vi "Operation DVR.vi"(8 "Error In":errorcluster, 11 "DVR In":refnum<data-value>) -> (0 "Error Out":errorcluster, 2 "C":dbl, 3 "DVR Out":refnum<data-value>)   [LabVIEW 2023, in "Arithemetic Operation.lvclass"]
uses:
  Arithemetic Operation.lvclass
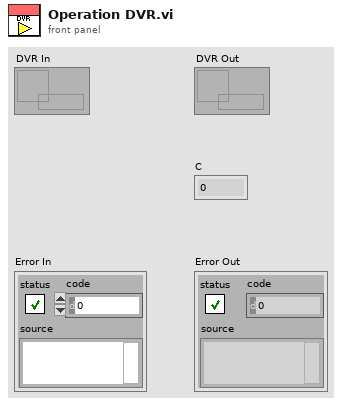
[diagram p1: front panel]
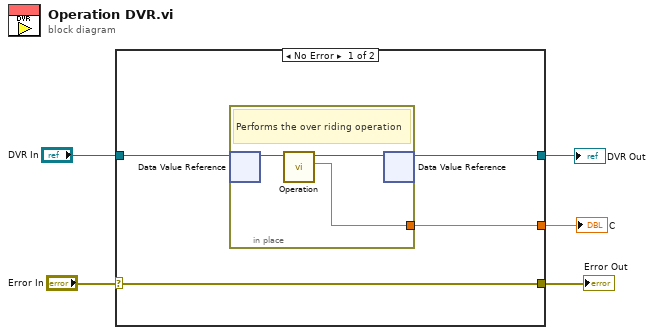
[diagram p0: block diagram]
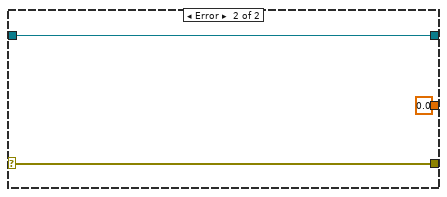
[diagram p2: hidden frame]
diagram:
  n1 = case shown="No Error" "Error In" {
    selector: "Error In" -> [w9 w15]
    tunnel: [w9 w15] -> w4
    tunnel: [w7 w14] -> w3
    tunnel: "DVR In" -> [w8 w14]
    tunnel: [w6 0.0 ("C")] -> w1
    frame No Error {
      n2 = in-place {
        in-place-border: [w10] -> w6
        # "Performs the over riding operation"
        n3 = in-place-dvr #1(w8) -> (w12:refnum<class "Arithemetic Operation.lvclass">)  [unwired: 1 out]
        n4 = call-dynamic "Operation.vi"("Arithemetic Operation in"=w12) -> ("C"=w10:dbl, "Arithemetic Operation out"=w11:refnum<class "Arithemetic Operation.lvclass">)  [unwired: 8 in, 1 out]
        n5 = in-place-dvr #1(w11) -> (w7:refnum<data-value>)  [unwired: 1 out]
      }
    }
    frame Error {
    }
  }
  "Error Out" <- w4
  "DVR Out" <- w3
  "C" <- w1
